vi "update.vi"(8 "error in (no error)":errorcluster, 11 "TrajectoryMG100122AODFrameScan in":refnum<class "TrajectoryMG100122AODFrameScan.lvclass">) -> (0 "error out":errorcluster, 3 "TrajectoryMG100122AODFrameScan out":refnum<class "TrajectoryMG100122AODFrameScan.lvclass">)   [LabVIEW 2010, in "TrajectoryMG100122AODFrameScan.lvclass"]
uses:
  TrajectoryMG100122AODFrameScan.lvclass
  FPGAWrapper/FPGAWrapperMH120124AOD/FPGAWrapperMH120124FrameScan_PXI7813R/FPGAWrapperMH120124FrameScan_PXI7813R.lvclass
  FPGAWrapper/GenericFPGAWrapper/GenericFPGAWrapper/GenericFPGAWrapper.lvclass
  common/classes/GenericComponent/GenericComponent/class_data.vi
  common/classes/GenericComponent/GenericComponent/GenericComponent.lvclass
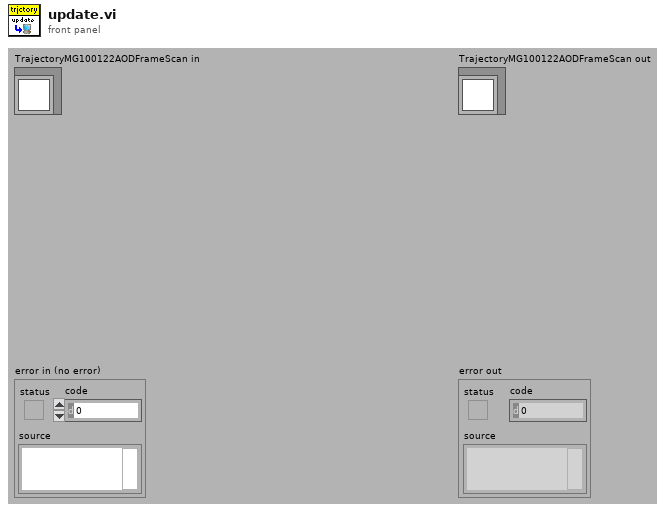
[diagram p1: front panel]
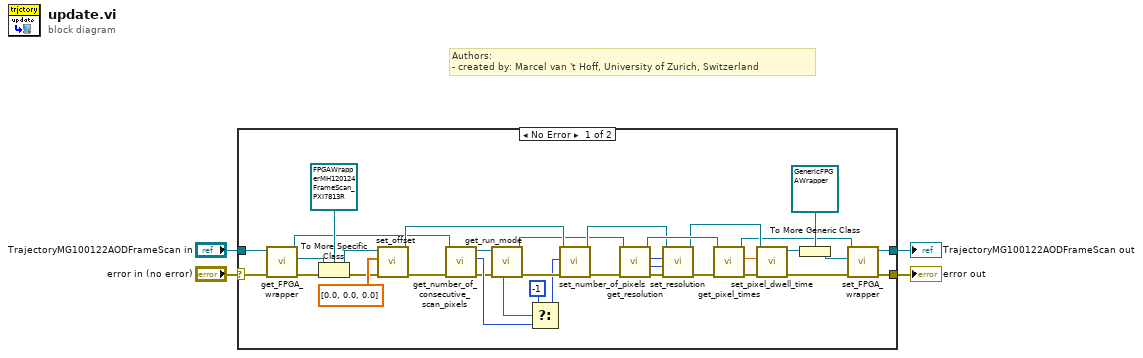
[diagram p0: block diagram]
diagram:
  # "Authors: \n- created by: Marcel van 't Hoff, University of Zurich, Switzerland"
  n1 = case shown="No Error" "error in (no error)" {
    selector: "error in (no error)" -> [w40 w42]
    tunnel: [w39 w42] -> w4
    tunnel: "TrajectoryMG100122AODFrameScan in" -> [w16 w41]
    tunnel: [w38 w41] -> w3
    frame No Error {
      n2 = call-dynamic "get_FPGA_wrapper.vi"("error in (no error)"=w40, "TrajectoryMG100122GenericFPGA in"=w16) -> ("error out"=w34:errorcluster, "GenericFPGAWrapper.lvclass"=w33:refnum<class "GenericFPGAWrapper.lvclass">, "TrajectoryMG100122GenericFPGA out"=w15:refnum<class "TrajectoryMG100122AODFrameScan.lvclass">)  [unwired: 7 in]
      n3 = To More Specific Class(target class=refnum<class "FPGAWrapperMH120124FrameScan_PXI7813R.lvclass"> refnum ("FPGAWrapperMH120124FrameScan_PXI7813R.lvclass"), reference=w33, error in=w34) -> (specific class reference=w8:refnum<class "FPGAWrapperMH120124FrameScan_PXI7813R.lvclass">, error out=w9:errorcluster)
      n4 = call-dynamic "set_offset.vi"("error in (no error)"=w9, "offset"=dbl[unit][] [0.0, 0.0, 0.0], "FPGAWrapperMH120124FrameScan_PXI7813R in"=w8) -> ("error out"=w13:errorcluster, "FPGAWrapperMH120124FrameScan_PXI7813R out"=w23:refnum<class "FPGAWrapperMH120124FrameScan_PXI7813R.lvclass">)  [unwired: 7 in]
      n5 = call-dynamic "get_number_of_consecutive_scan_pixels.vi"("error in (no error)"=w13, "GenericTrajectory in"=w15) -> ("error out"=w17:errorcluster, "number of consecutive scan pixels"=w20:i64, "GenericTrajectory out"=w18:refnum<class "TrajectoryMG100122AODFrameScan.lvclass">)  [unwired: 7 in]
      n6 = call "get_run_mode.vi"("error in (no error)"=w17, "GenericPlugin in"=w18) -> ("error out"=w14:errorcluster, "GenericPlugin out"=w11:refnum<class "TrajectoryMG100122AODFrameScan.lvclass">, "is free run?"=w21:bool)  [unwired: 5 in, 2 out]
      n7 = Select(t=i64 -1, s=w21, f=w20) -> (s? t:f=w10:i64)
      n8 = call-dynamic "set_number_of_pixels.vi"("error in (no error)"=w14, "number of pixels"=w10, "FPGAWrapperMH120124FrameScan_PXI7813R in"=w23) -> ("error out"=w12:errorcluster, "FPGAWrapperMH120124FrameScan_PXI7813R out"=w22:refnum<class "FPGAWrapperMH120124FrameScan_PXI7813R.lvclass">)  [unwired: 7 in]
      n9 = call-dynamic "get_resolution.vi"("error in (no error)"=w12, "TrajectoryMG100122AODFrameScan in"=w11) -> ("error out"=w30:errorcluster, "y resolution"=w27:i32, "x resolution"=w28:i32, "TrajectoryMG100122AODFrameScan out"=w35:refnum<class "TrajectoryMG100122AODFrameScan.lvclass">)  [unwired: 6 in]
      n10 = call-dynamic "set_resolution.vi"("error in (no error)"=w30, "y resolution"=w27, "x resolution"=w28, "FPGAWrapperMH120124FrameScan_PXI7813R in"=w22) -> ("error out"=w29:errorcluster, "FPGAWrapperMH120124FrameScan_PXI7813R out"=w26:refnum<class "FPGAWrapperMH120124FrameScan_PXI7813R.lvclass">)  [unwired: 6 in]
      n11 = call-dynamic "get_pixel_times.vi"("error in (no error)"=w29, "TrajectoryMG100122AODFrameScan in"=w35) -> ("error out"=w25:errorcluster, "acquisition time"=w24:dbl[unit], "TrajectoryMG100122AODFrameScan out"=w7:refnum<class "TrajectoryMG100122AODFrameScan.lvclass">)  [unwired: 5 in, 2 out]
      n12 = call-dynamic "set_pixel_dwell_time.vi"("error in (no error)"=w25, "pixel dwell time"=w24, "FPGAWrapperMH120124FrameScan_PXI7813R in"=w26) -> ("error out"=w6:errorcluster, "FPGAWrapperMH120124FrameScan_PXI7813R out"=w5:refnum<class "FPGAWrapperMH120124FrameScan_PXI7813R.lvclass">)  [unwired: 7 in]
      n13 = To More Generic Class(target class=refnum<class "GenericFPGAWrapper.lvclass"> refnum ("GenericFPGAWrapper.lvclass"), reference=w5) -> (generic class reference=w36:refnum<class "GenericFPGAWrapper.lvclass">)
      n14 = call-dynamic "set_FPGA_wrapper.vi"("error in (no error)"=w6, "GenericFPGAWrapper.lvclass"=w36, "TrajectoryMG100122GenericFPGA in"=w7) -> ("error out"=w39:errorcluster, "TrajectoryMG100122GenericFPGA out"=w38:refnum<class "TrajectoryMG100122AODFrameScan.lvclass">)  [unwired: 7 in]
    }
    frame Error {
    }
  }
  "error out" <- w4
  "TrajectoryMG100122AODFrameScan out" <- w3
